vi "Create Song Library.vi"(8 "error in (no error)":errorcluster, 9 "Songs":refnum<class "Song.lvclass">[](array[class]), 10 "Name":string, 11 "SongLibrary In":refnum<class "SongLibrary.lvclass">) -> (0 "error out":errorcluster, 3 "SongLibrary out":refnum<class "SongLibrary.lvclass">)   [LabVIEW 2015, in "SongLibrary.lvclass"]
uses:
  SongLibrary.lvclass
  Song/Song.lvclass
  MusicElementLibrary.lvclass
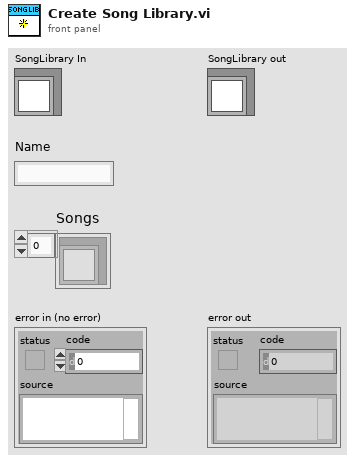
[diagram p1: front panel]
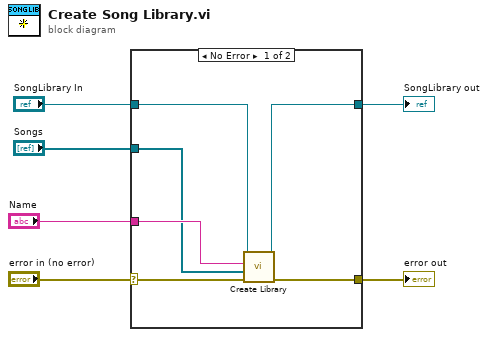
[diagram p0: block diagram]
diagram:
  n1 = case shown="No Error" "error in (no error)" {
    selector: "error in (no error)" -> [w9 w14]
    tunnel: [w12 w14] -> w5
    tunnel: [w10 w13] -> w4
    tunnel: "SongLibrary In" -> [w11 w13]
    tunnel: "Name" -> [w8 _]
    tunnel: "Songs" -> [w7 _]
    frame No Error {
      n2 = call "Create Library.vi"("error in (no error)"=w9, "Music Element Library"=w7, "Name"=w8, "MusicElementLibrary in"=w11) -> ("error out"=w12:errorcluster, "MusicElementLibrary out"=w10:refnum<class "SongLibrary.lvclass">)  [unwired: 6 in]
    }
    frame Error {
    }
  }
  "error out" <- w5
  "SongLibrary out" <- w4
